vi "XSP3_PutString(1D).vi"(6 "String":string, 8 "ErrorIn":errorcluster, 9 "Time":dbl=1.0 caption="TimeOut/s", 10 "Wait":u32=10 caption="Wait/ms", 11 "PVIn":string caption="PVNameIn") -> (0 "ErrorOut":errorcluster, 2 "Status":bool, 3 "PVOut":string caption="PVNameOut", 4 "PVError":errorcluster)   [LabVIEW 2010]
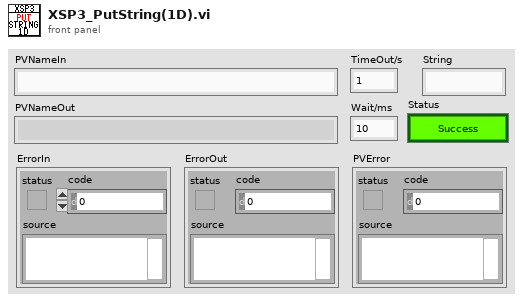
[diagram p1: front panel]
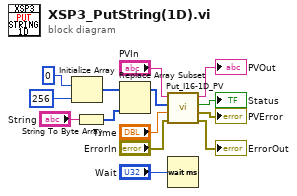
[diagram p0: block diagram]
diagram:
  n1 = Initialize Array(i16 0, 256 ("次元サイズ")) -> (w13:i16[])
  n2 = String To Byte Array(string="String") -> (unsigned byte array=w11:u8[])
  n3 = Replace Array Subset(array=w13, new element=w11) -> (w10:i16[])  [unwired: 1 in]
  n4 = call "Put_I16-1D_PV.vi"("Error in (no error)"="ErrorIn", "Timeout (3)"="Time", "Values"=w10, "PV Name"="PVIn") -> ("Error out"=→"ErrorOut":errorcluster, "PV error"=→"PVError":errorcluster, "Status"=→"Status":bool, "PV Name (dup)"=→"PVOut":string)  [unwired: 4 in]
  n5 = Wait (ms)(milliseconds to wait="Wait") -> ()  [unwired: 1 out]
